vi "Pre Launch Init.vi"(11 "Jobber Proxy in":refnum<class "Jobber Proxy.lvclass">) -> (0 "error out":errorcluster, 3 "Jobber Proxy out":refnum<class "Jobber Proxy.lvclass">)   [LabVIEW 2014, in "Jobber Proxy.lvlib" / "Jobber Proxy.lvclass"]
doc: "(<B>Filename</B>: Actor Framework.lvlib:Actor.lvclass:Pre Launch Init.vi)\n\nDefines behavior that occurs after the Launch Nested Actor method is invoked but before the actor's Actor Core method begins running.\n\nBy default, this method does nothing. A descendant class may override it to define behavior."
uses:
  Jobber Proxy.lvclass
  Jobber Proxy.lvclass/Jobber Proxy.ctl
  <vilib>/ActorFramework/Actor/Actor.lvclass
  Classes/LabVIEW Instance/LabVIEW Instance.lvclass
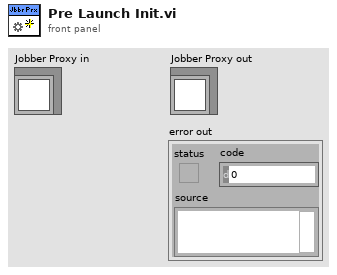
[diagram p1: front panel]
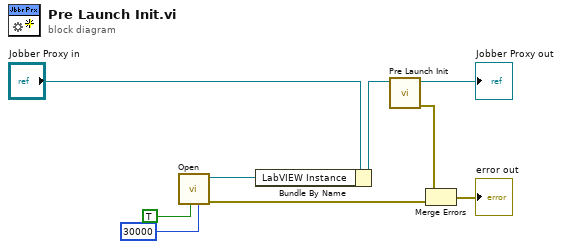
[diagram p0: block diagram]
diagram:
  n1 = call "Open.vi"("Wait"=u32 30000, "Show Panel"=TRUE) -> ("error out"=w1:errorcluster, "LabVIEW Instance"=w3:refnum<class "LabVIEW Instance.lvclass">)  [unwired: 8 in]
  n2 = Bundle By Name(cluster="Jobber Proxy in", "LabVIEW Instance"=w3) -> (w6:refnum<class "Jobber Proxy.lvclass">)
  n3 = call-parent "Pre Launch Init.vi"("Actor in"=w6) -> ("error out"=w9:errorcluster, "Actor out"=→"Jobber Proxy out":refnum<class "Jobber Proxy.lvclass">)  [unwired: 9 in]
  n4 = Merge Errors(w9, w1) -> (→"error out":errorcluster)
